vi "180 Wrap.vi"(10 "yawOffset":dbl, 11 "Yaw":dbl) -> (3 "Numeric":dbl)   [LabVIEW 2019]
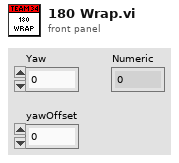
[diagram p1: front panel]
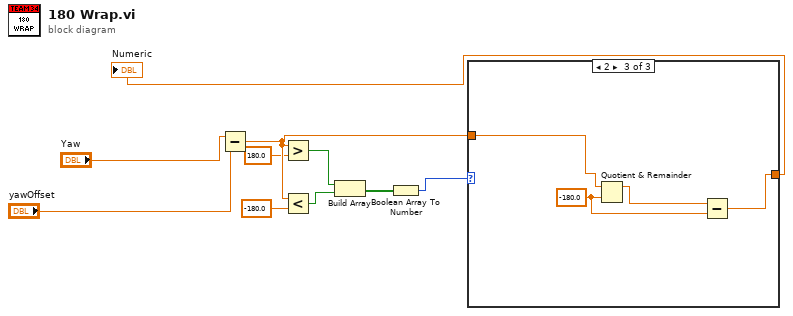
[diagram p0: block diagram]
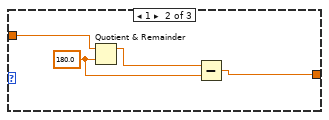
[diagram p3: hidden frame]
diagram:
  n1 = Subtract(x="Yaw", y="yawOffset") -> (x-y=w7:dbl)
  n2 = Greater?(x=w7, y=180.0) -> (0:w3:bool)
  n3 = Less?(x=w7, y=-180.0) -> (x < y?=w4:bool)
  n4 = Build Array(w3, w4) -> (w5:bool[])
  n5 = Boolean Array To Number(Boolean array=w5) -> (number=w6:u32)
  n6 = case shown="2" w6 {
    tunnel: [w11 w13 w17] -> w8
    tunnel: w7 -> [w11 w12 w16]
    frame 0, Default {
    }
    frame 1 {
      w14 = 180.0 ("y")
      n7 = Quotient & Remainder(x=w12, y=w14) -> (x-y*floor(x/y)=w15:dbl)  [unwired: 1 out]
      n8 = Subtract(x=w15, y=w14) -> (x-y=w13:dbl)
    }
    frame 2 {
      w18 = -180.0 ("y")
      n9 = Quotient & Remainder(x=w16, y=w18) -> (x-y*floor(x/y)=w19:dbl)  [unwired: 1 out]
      n10 = Subtract(x=w19, y=w18) -> (x-y=w17:dbl)
    }
  }
  "Numeric" <- w8
